vi "Get Curve Limitation.vi"(8 "error in (no error)":errorcluster, 11 "ProductNum":string) -> (0 "error out":errorcluster, 1 "X data Range":dbl[](array[numeric]), 2 "Kb":T1, 3 "Up down Limit XY array":cluster{dbl[], "Xt resampled":dbl[]}[](array[cluster]))   [LabVIEW 2015, in "SQLite.lvclass"]
doc: "写入每一步的测试结果到Results表格。\n写入原理：先检测已经保存了几个结果数据，然后依次附加到结果数据列上。\n# 2020-6-8 14:05:45"
uses:
  SQLite.lvclass
  TwoPoint Curve Limitation Kb.ctl
  SQLiteFileName.ctl
  TabelFullName.ctl
  <vilib>/Utility/error.llb/Trim Whitespace.vi
  <vilib>/addons/Time Series Analysis/Series Preprocess.llb/TSA Resampling (Equal).vi
  <userlib>/sushu/sushu.lvlib
  <vilib>/addons/_Advanced Signal Processing/NI_AdvSigProcTSA.lvlib
panel:
  out "XY Graph":cluster{dbl[], dbl[]}[](graph)
  out "appended array 2":dbl[](array[numeric])
  out "appended array":dbl[](array[numeric])
  in  "Results List":string
  out "CMD":string
  in  "StationName":string
  out "number (0 to 1)":dbl
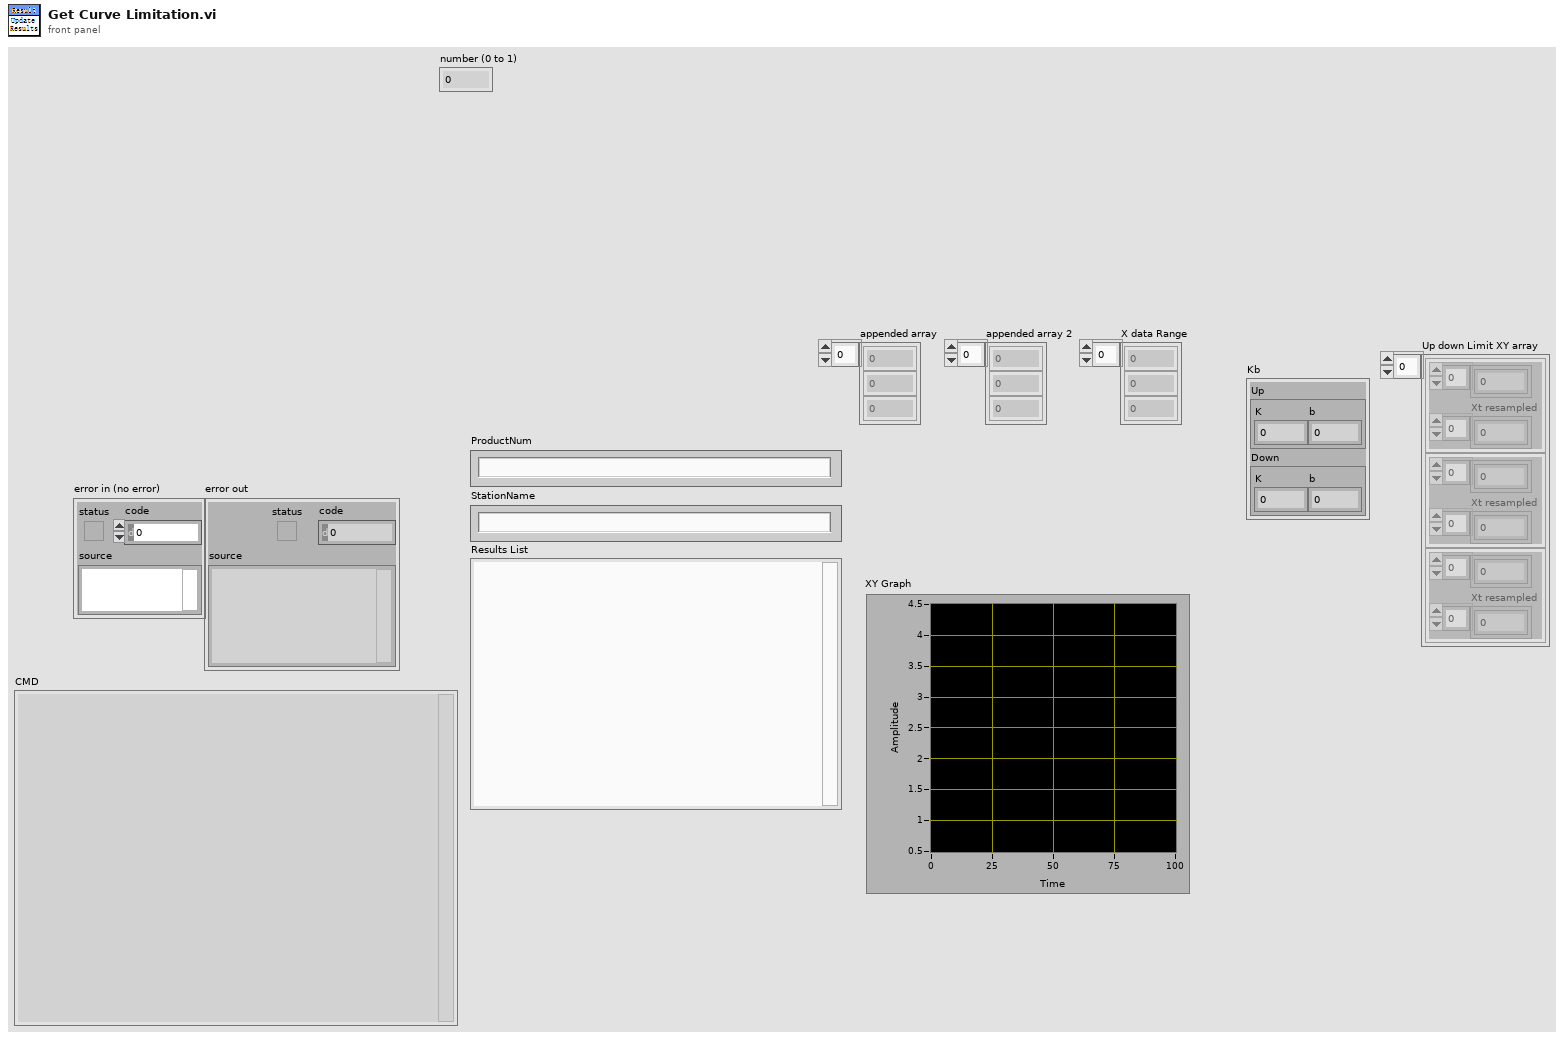
[diagram p1: front panel]
types:
  T1 = typedef "SQLite.lvclass/TwoPoint Curve Limitation Kb.ctl" = cluster{"Up":cluster{"K":dbl, "b":dbl}, "Down":cluster{"K":dbl, "b":dbl}}
  T2 = typedef "SQLite.lvclass/TabelFullName.ctl" = string
  T3 = typedef "SQLite.lvclass/SQLiteFileName.ctl" = string
  T4 = cluster{"Core":cluster{"Current VI Reference":refnum<vi>, "Close Panel on Exit?":bool}, "VI Name":string, "Row Numbers":string, "Update?":bool, "CMD":string, "ResultStartindex":i32, "EmptyResultColumnIndex":i32, "Kb":T1}
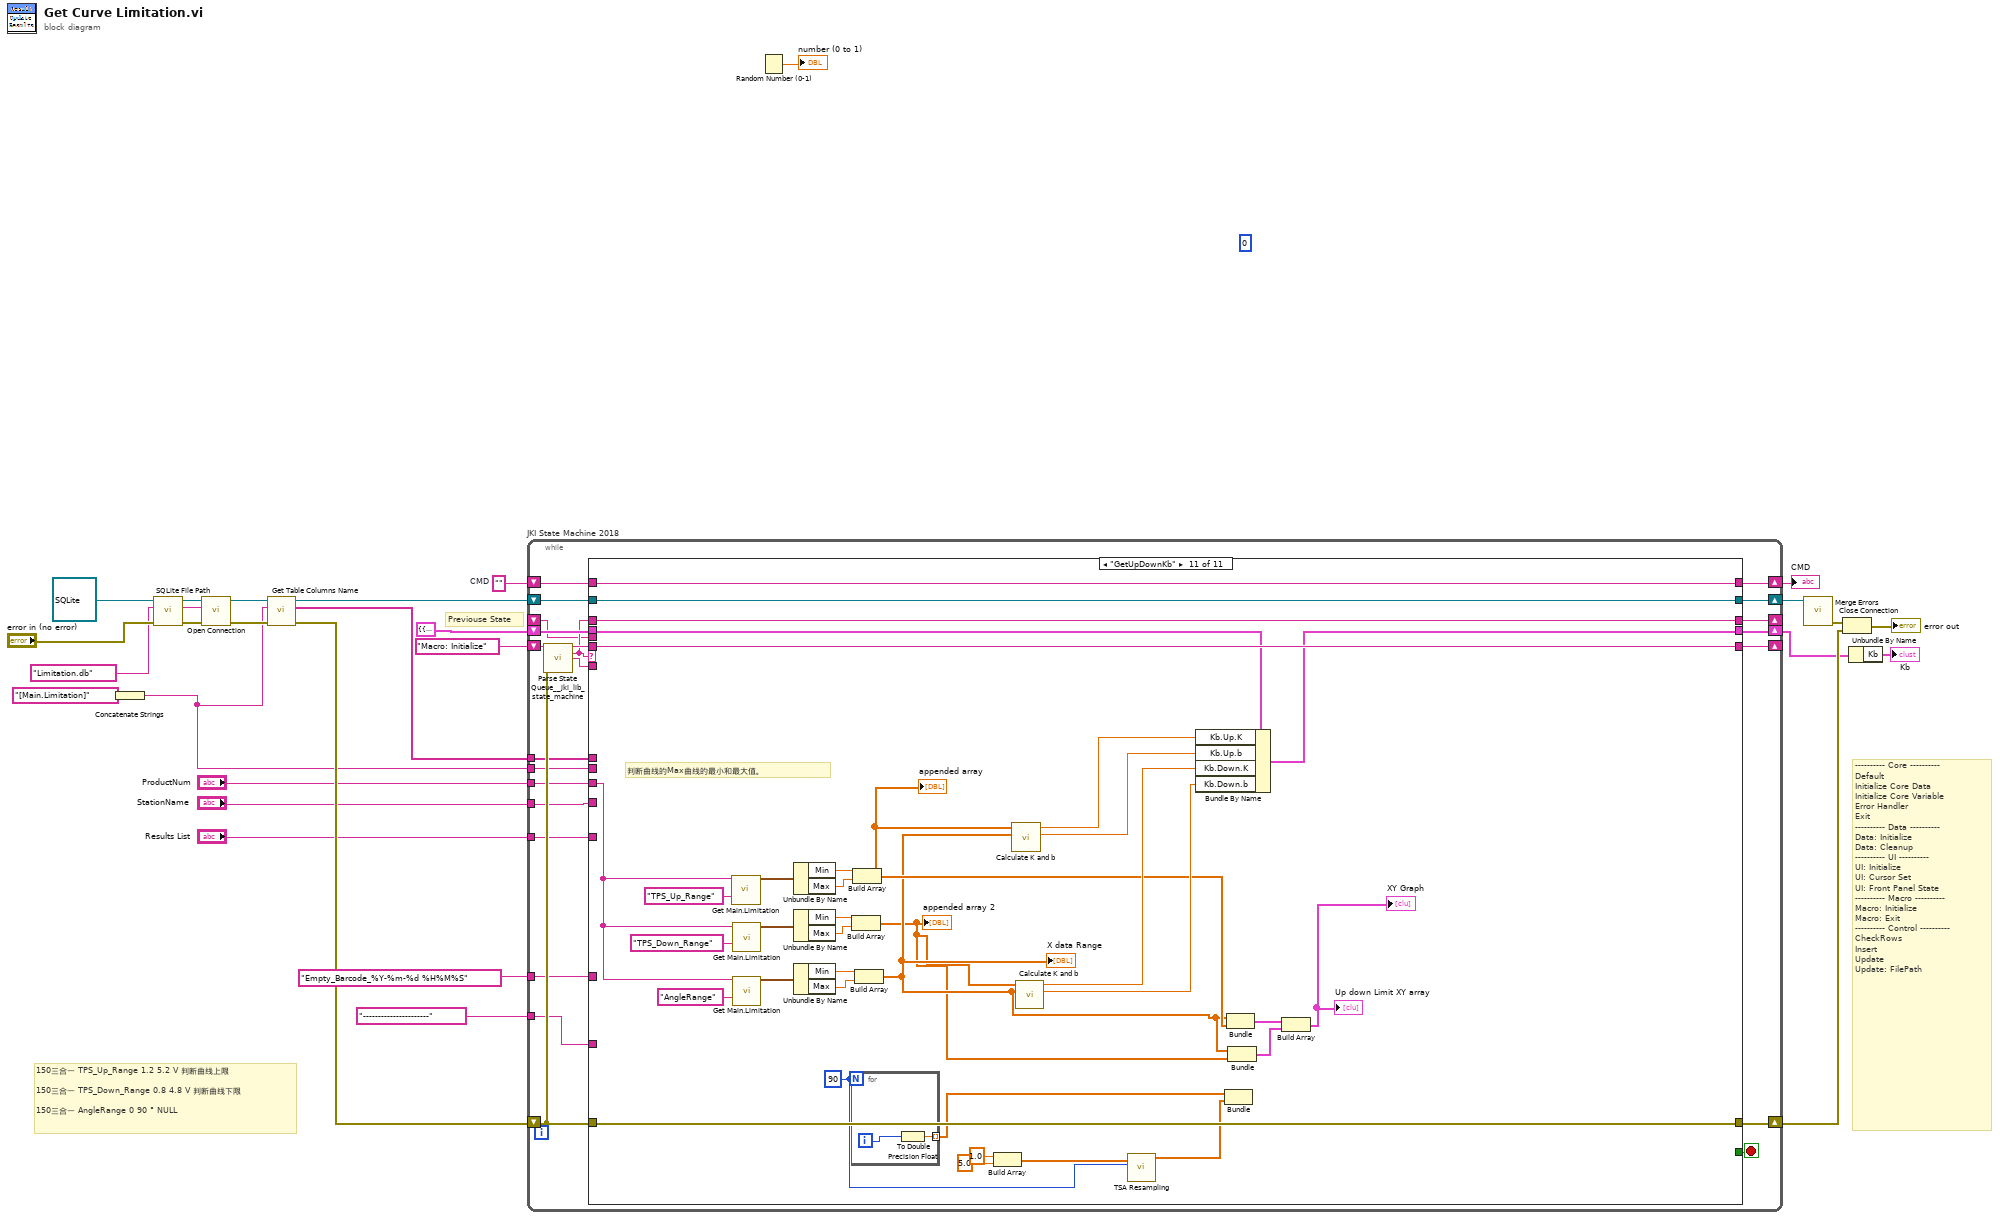
[diagram p0: block diagram]
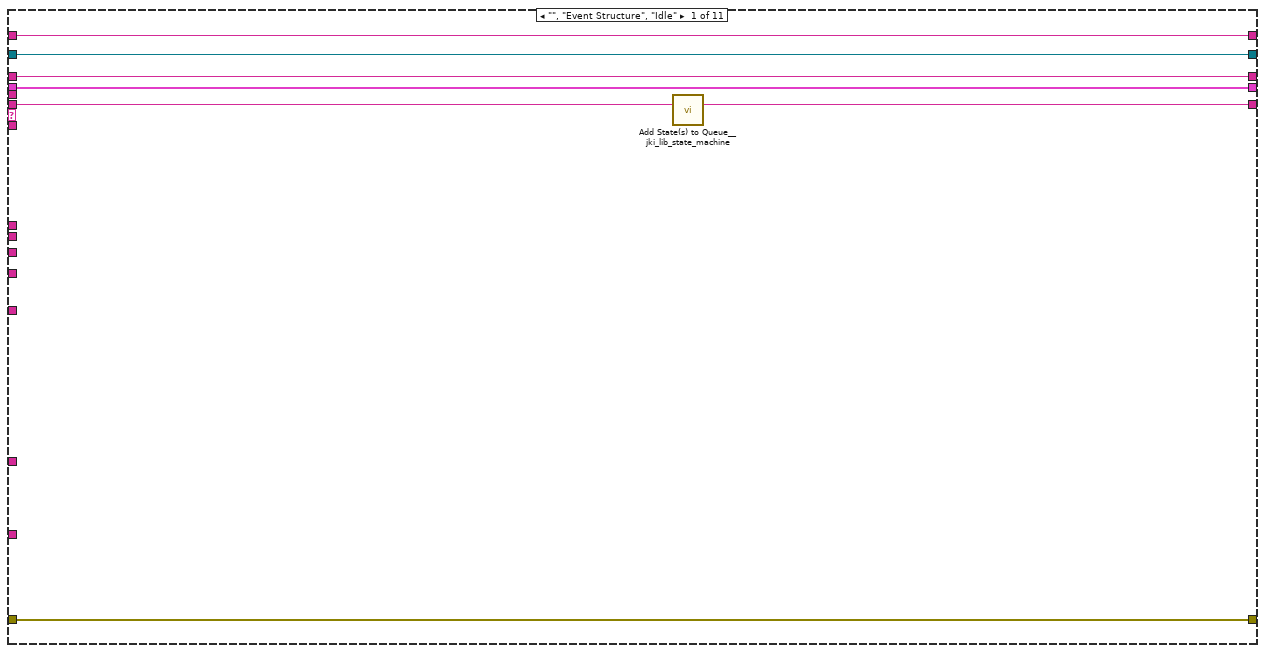
[diagram p2: hidden frame]
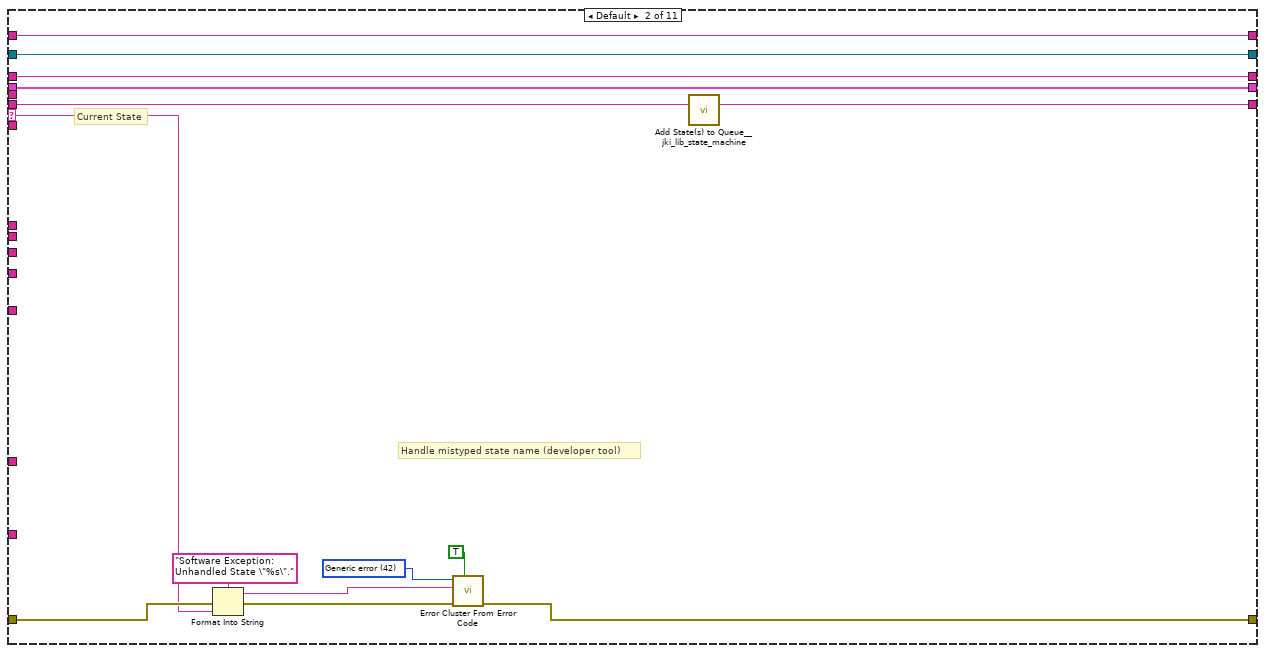
[diagram p3: hidden frame]
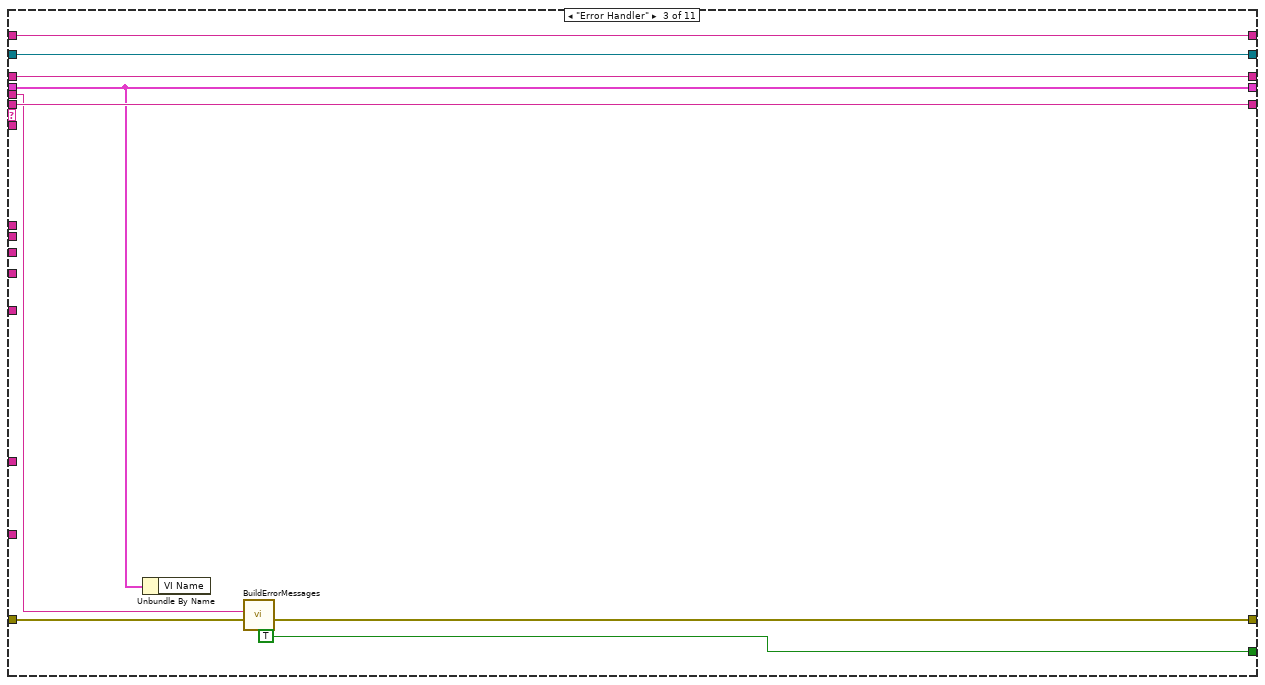
[diagram p4: hidden frame]
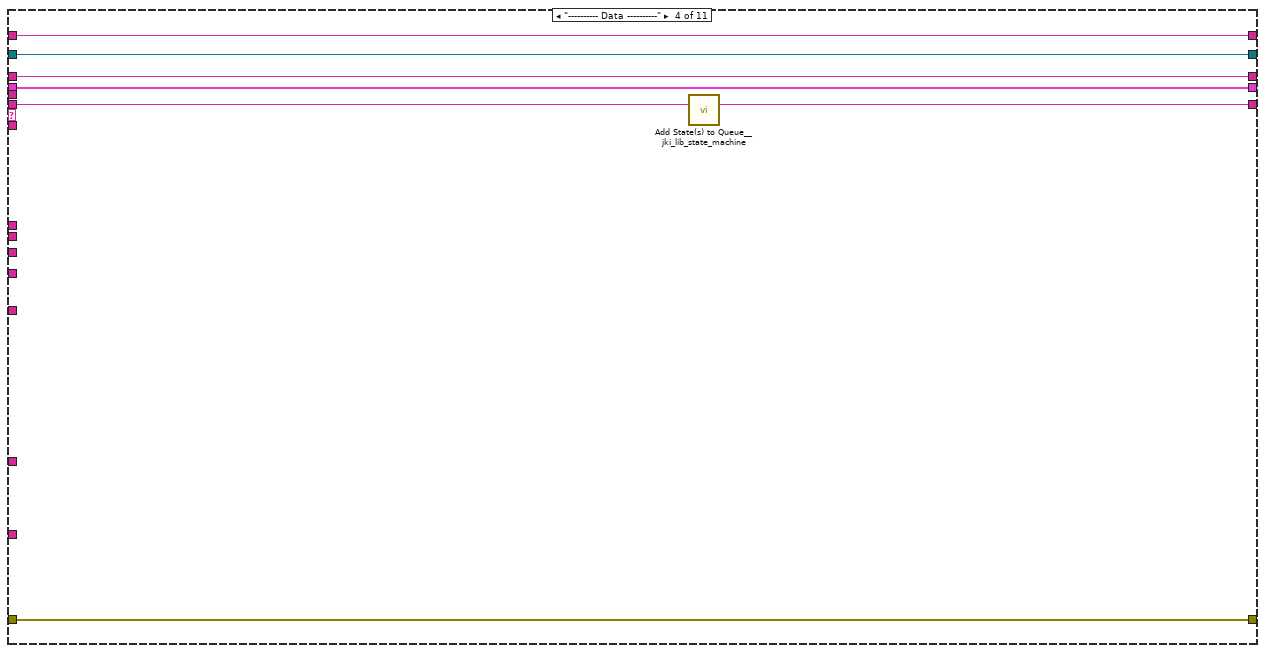
[diagram p5: hidden frame]
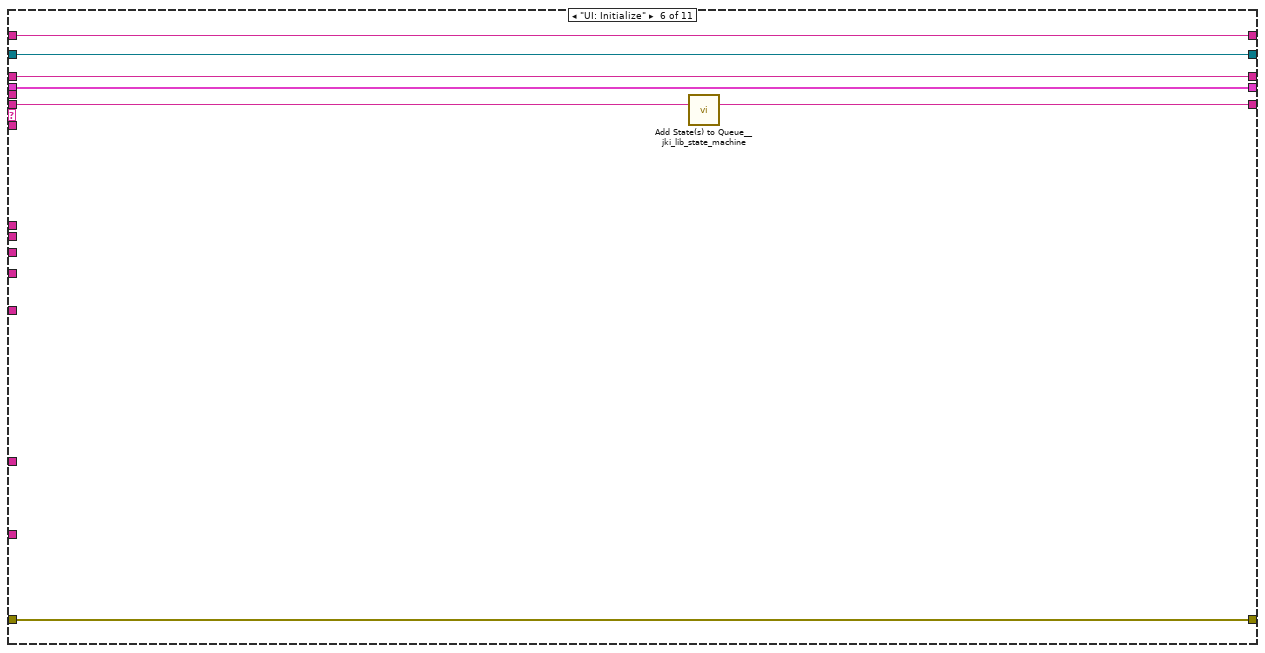
[diagram p7: hidden frame]
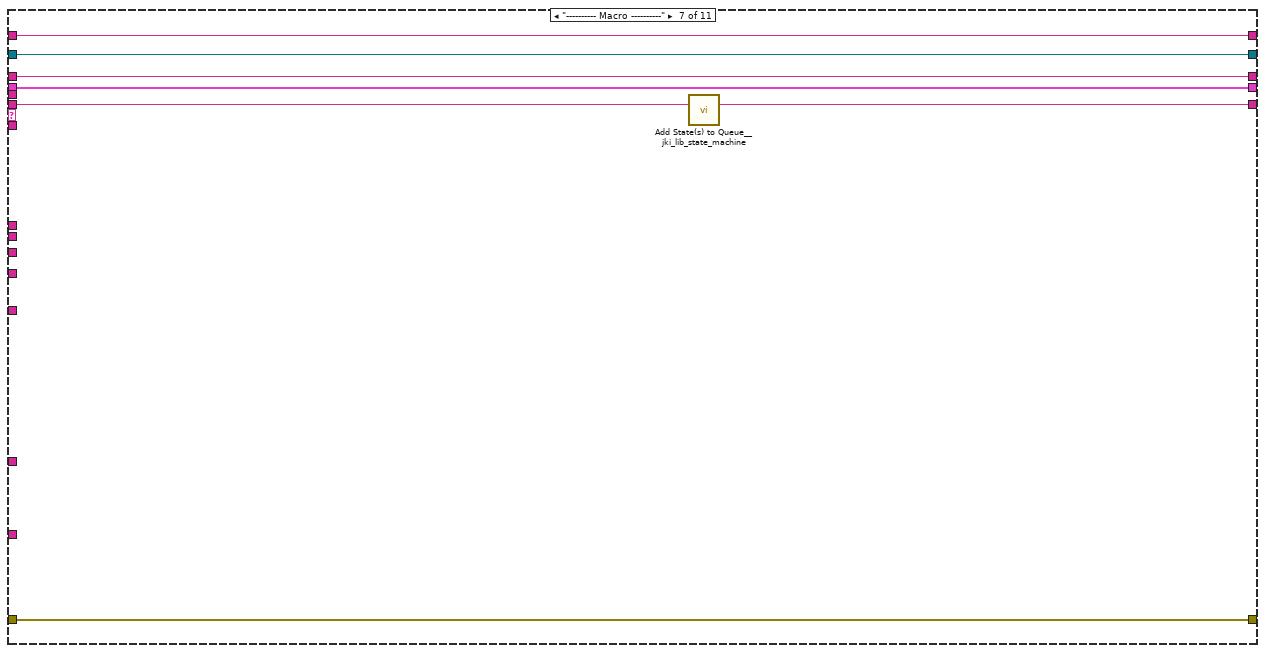
[diagram p8: hidden frame]
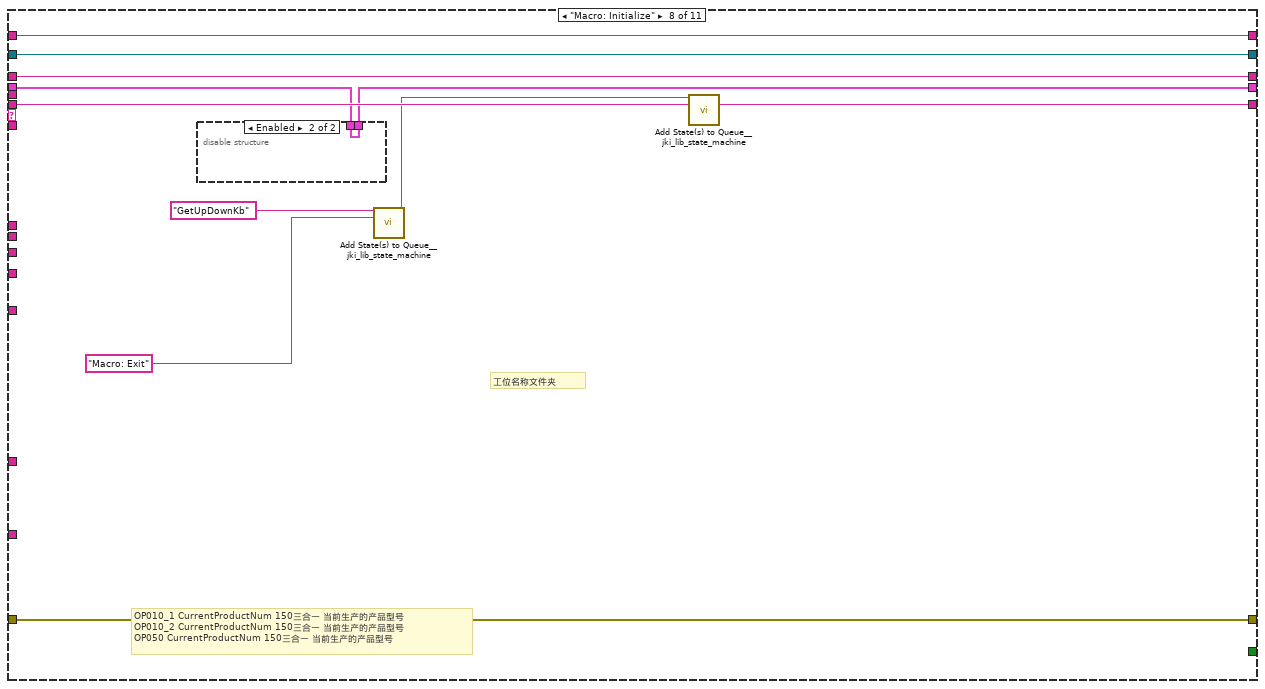
[diagram p9: hidden frame]
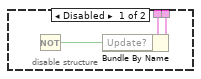
[diagram p10: hidden frame]
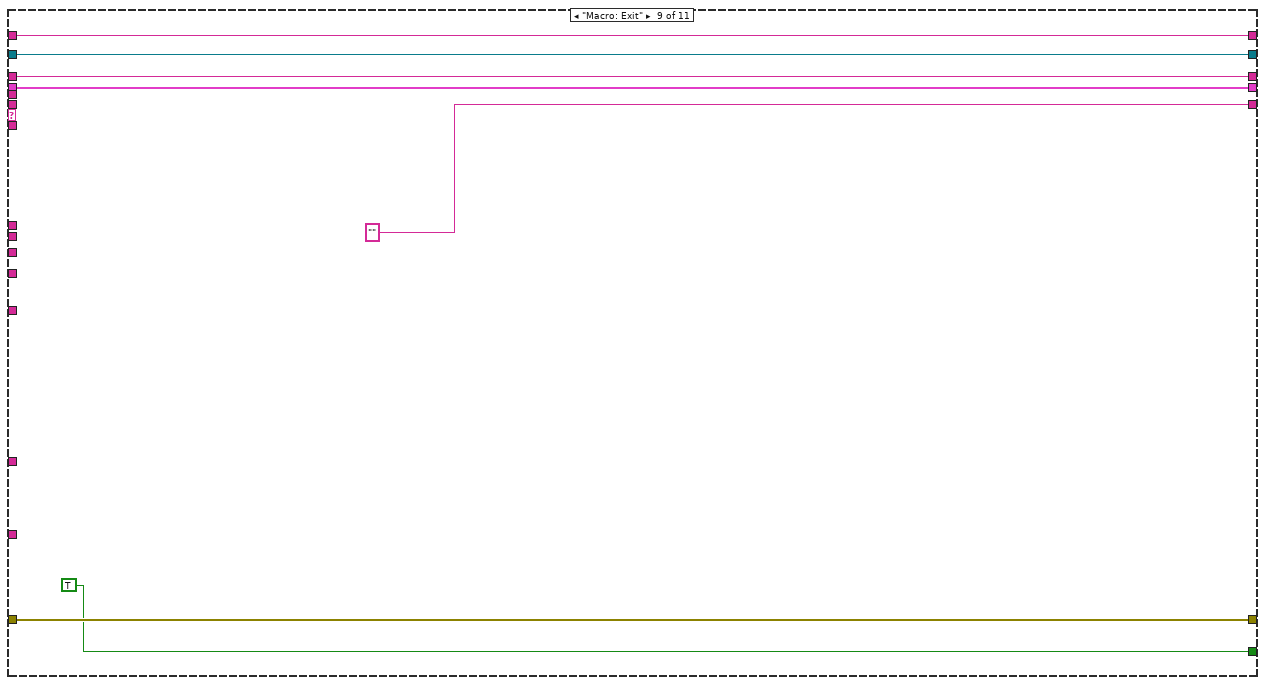
[diagram p11: hidden frame]
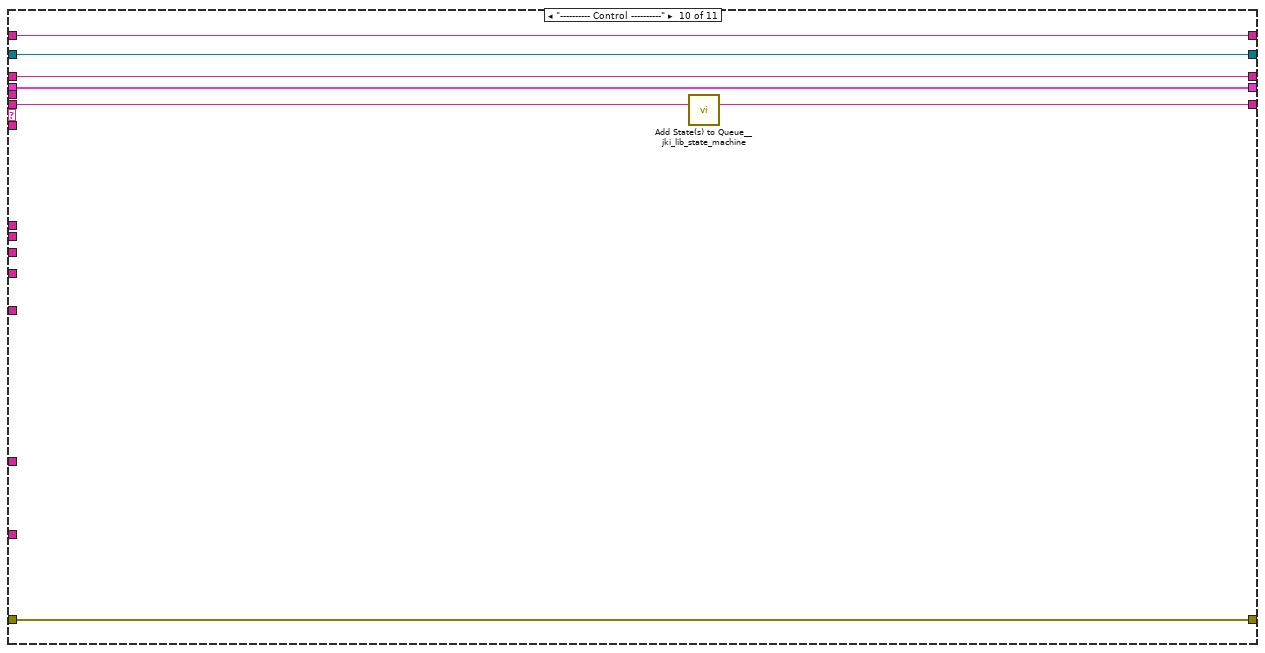
[diagram p12: hidden frame]
diagram:
  w14 = ""  # CMD
  (unwired) 0 ("index (row)")
  # "150三合一\tTPS_Up_Range\t1.2\t5.2\tV\t判断曲线上限\n\n150三合一\tTPS_Down_Range\t0.8\t4.8\tV\t判断曲线下限\n\n150三合一\tAngleRange\t0\t90\t°\tNULL"
  # "Previouse State"
  # "---------- Core ----------\nDefault\nInitialize Core Data\nInitialize Core Variable\nError Handler\nExit\n---------- Data ----------\nData: Initialize\nData: Cleanup\n---------- UI ----------\nUI: Initialize\nUI: Cursor Set\nUI: Front Panel State\n---------- Macro ----------\nMacro: Initialize\nMacro: Exit\n---------- Control ----------\nCheckRows\nInsert\nUpdate\nUpdate: FilePath"
  n1 = Concatenate Strings(T2 "[Main.Limitation]" ("TabelFullName")) -> (w3:string)
  n2 = call "SQLite File Path.vi"("error in (no error)"="error in (no error)", "SQLiteFileName"=T3 "Limitation.db", "SQLite in"=refnum<class "SQLite.lvclass"> refnum ("SQLite.lvclass")) -> ("error out"=w6:errorcluster, "string"=w10:string, "SQLite out"=w8:refnum<class "SQLite.lvclass">)  [unwired: 6 in]
  n3 = call-dynamic "Open Connection.vi"("error in (no error)"=w6, "ConnectionString"=w10, "HostDB in"=w8) -> ("error out"=w27:errorcluster, "HostDB out"=w28:refnum<class "SQLite.lvclass">)  [unwired: 7 in]
  n4 = call-dynamic "Get Table Columns Name.vi"("error in (no error)"=w27, "TableName"=w3, "HostDB in"=w28) -> ("error out"=w19:errorcluster, "ColunmsList"=w18:string[], "HostDB out"=w23:refnum<class "SQLite.lvclass">)  [unwired: 4 in, 2 out]
  n5 = while "JKI State Machine 2018" {
    shift-right: [w46] -> w2
    shift-left: T4 {"Core"={"Current VI Reference"=refnum, "Close Panel on Exit?"=FALSE}, "VI Name"="", "Row Numbers"="", "Update?"=FALSE, "CMD"="", "ResultStartindex"=0, "EmptyResultColumnIndex"=0, "Kb"={"Up"={"K"=0.0, "b"=0.0}, "Down"={"K"=0.0, "b"=0.0}}} ("Data") -> [w45]
    shift-right: [w49] -> w20
    shift-left: w19 -> [w44]
    shift-right: [w48] -> _
    shift-left: "Macro: Initialize" -> [w50]
    shift-right: [w42] -> w22
    shift-left: w23 -> [w43]
    shift-right: [w40] -> _
    shift-left: _ -> [w39]
    tunnel: "StationName" -> [w38]
    tunnel: "ProductNum" -> [w37]
    tunnel: w18 -> [w36]
    tunnel: w3 -> [w35]
    tunnel: "Empty_Barcode_%Y-%m-%d %H%M%S" ("time format string (%c)") -> [w34]
    shift-right: [w33] -> w12
    shift-left: w14 -> [w32]
    tunnel: "----------------------" ("State(s) in (\"\")") -> [w31]
    tunnel: "Results List" -> [w30]
    stop <- w47 stop-if-true
    n6 = call <vilib>:"Parse State Queue__jki_lib_state_machine.vi"("State Queue"=w50, "Error In (no error)"=w44) -> ("Remaining States"=w52:string, "Current State"=w41:string, "Arguments"=w51:string)  [unwired: 11 in]
    n7 = case shown="\"GetUpDownKb\"" w41 {
      selector: w41 -> [_ w63 _ _ _ _ _ _ _ _ _]
      tunnel: w52 -> [w59 w67 w81 w89 w92 w102 w109 w120 _ w138 w173]
      tunnel: w51 -> [_ _ _ _ _ _ _ _ _ _ _]
      tunnel: w45 -> [w56 w65 w78 w86 w93 w100 w106 w115 w130 w135 w152]
      tunnel: [w57 w69 w75 w87 w95 w99 w107 w116 w131 w136 w174] -> w49
      tunnel: w44 -> [w57 w68 w76 w87 w95 w99 w107 w116 w131 w136 w174]
      tunnel: [w58 w66 w81 w88 w92 w101 w108 w119 "" w137 w173] -> w48
      tunnel: [_ _ TRUE _ _ _ _ _ TRUE _ _] -> w47
      tunnel: [w56 w65 w78 w86 w93 w100 w106 w111 w130 w135 w151] -> w46
      tunnel: w43 -> [w55 w62 w80 w85 w94 w98 w105 w118 w129 w134 w172]
      tunnel: [w55 w62 w80 w85 w94 w98 w105 w118 w129 w134 w172] -> w42
      tunnel: w41 -> [w54 w61 w79 w84 w91 w97 w104 w117 w127 w133 w171]
      tunnel: [w54 w61 w79 w84 w91 w97 w104 w117 w127 w133 w171] -> w40
      tunnel: w39 -> [_ _ w77 _ _ _ _ _ _ _ _]
      tunnel: w38 -> [_ _ _ _ _ _ _ _ _ _ _]
      tunnel: w37 -> [_ _ _ _ _ _ _ _ _ _ w166]
      tunnel: w36 -> [_ _ _ _ _ _ _ _ _ _ _]
      tunnel: w35 -> [_ _ _ _ _ _ _ _ _ _ _]
      tunnel: w34 -> [_ _ _ _ _ _ _ _ _ _ _]
      tunnel: w32 -> [w53 w60 w74 w83 w90 w96 w103 w112 w125 w132 w170]
      tunnel: [w53 w60 w74 w83 w90 w96 w103 w112 w125 w132 w170] -> w33
      tunnel: w31 -> [_ _ _ _ _ _ _ _ _ _ _]
      tunnel: w30 -> [_ _ _ _ _ _ _ _ _ _ _]
      frame "", "Event Structure", "Idle" {
        n8 = call <vilib>:"Add State(s) to Queue__jki_lib_state_machine.vi"("State(s) in (\"\")"=w59) -> ("States Out"=w58:string)  [unwired: 14 in]
      }
      frame Default {
        w72 = 42 items=["No error", "Argument error", "Memory is full", "Out of zone", "End of file", "File already open", "Generic file I/O error", "File not found", "File permission error", "Disk is full", "Duplicate path", "Too many files open", "System feature not enabled", "Resource file not found", "Cannot add resource", "Resource not found", "Image not found", "Image memory error", "Pen does not exist", "Config type invalid", "Config token not found", "Config parse error", "Config memory error", "Bad external code format", "Bad external code offset", "External code not present", "Null window", "Destroy window error", "Null menu", "Print aborted", "Bad print record", "Print driver error", "Windows error during printing", "Memory error during printing", "Print dialog error", "Generic print error", "Invalid device refnum", "Device not found", "Device parameter error", "Device unit error", "Cannot open device", "Device call aborted", "Generic error", "Cancelled by user", "Object ID too low", "Object ID too high", "Object not in heap", "Unknown heap", "Unknown object (invalid DefProc)", "Unknown object (DefProc not in table)", "Message out of range", "Invalid (null) method", "Unknown message", "Manager call not supported", "Bad address", "Network operation in progress", "Network operation timed out", "Connection is busy", "Network attribute not supported", "Network error", "Address in use", "System out of memory", "Connection aborted", "Connection refused", "Not connected", "Already connected", "Connection closed", "Initialization error (interapplication manager)", "Bad occurrence", "Wait on unbound occurrence handler", "Occurrence queue overflow", "Datalog type conflict", "Unused", "Unrecognized type (interapplication manager)", "Memory corrupt", "Failed to make temporary DLL", "Old CIN version", "Drag socket not found", "Failed to load drop-object", "Failed to register OLE object", "Failed to release OLE object", "Format specifier type mismatch", "Unknown format specifier", "Too few format specifiers", "Too many format specifiers", "Scan failed", "Newer CIN version", "Error converting to variant", "Runtime menu error", "Password tampered", "Variant attribute not found", "Incompatible variant data type", "Event data is not available", "Event Store is not present", "Occurrence is not found", "Event Queue is not created", "Event info is not available", "Refnum passed is NULL", "Error retrieving Class GUID", "Error retrieving CoClass GUID", "Error retrieving TypeLib GUID.", "Bad built application magic bytes.", "Specific driver is different from the specific driver associated with the Logical Name.", "There is no session opened to the class driver.", "Max Error", "MAX - Error with config objects", "MAX - Error loading configuration", "MAX - Group not supported"]
        # "Current State"
        # "Handle mistyped state name (developer tool)"
        n9 = Format Into String(format string="Software Exception: Unhandled State \"%s\"." ("message"), error in=w68, w63) -> (resulting string=w71:string, error out=w70:errorcluster)  [unwired: 1 in]
        n10 = call <vilib>:"Error Cluster From Error Code.vi"("show call chain? (False)"=TRUE, "error in (no error)"=w70, "error message (\"\")"=w71, "error code (0)"=w72) -> ("error out"=w69:errorcluster)  [unwired: 5 in]
        n11 = call <vilib>:"Add State(s) to Queue__jki_lib_state_machine.vi"("State(s) in (\"\")"=w67) -> ("States Out"=w66:string)  [unwired: 14 in]
      }
      frame "Error Handler" {
        n12 = Unbundle By Name(w78) -> ()  [unwired: 1 out]
        n13 = call <userlib>:"BuildErrorMessages.vi"("error in"=w76, "ErrorCase"=w77) -> ("error out (no error)"=w75:errorcluster)  [unwired: 7 in, 2 out]
      }
      frame "---------- Data ----------" {
        n14 = call <vilib>:"Add State(s) to Queue__jki_lib_state_machine.vi"("State(s) in (\"\")"=w89) -> ("States Out"=w88:string)  [unwired: 14 in]
      }
      frame "Data: Initialize" {
      }
      frame "UI: Initialize" {
        n15 = call <vilib>:"Add State(s) to Queue__jki_lib_state_machine.vi"("State(s) in (\"\")"=w102) -> ("States Out"=w101:string)  [unwired: 14 in]
      }
      frame "---------- Macro ----------" {
        n16 = call <vilib>:"Add State(s) to Queue__jki_lib_state_machine.vi"("State(s) in (\"\")"=w109) -> ("States Out"=w108:string)  [unwired: 14 in]
      }
      frame "Macro: Initialize" {
        # "OP010_1\tCurrentProductNum\t150三合一\t当前生产的产品型号\nOP010_2\tCurrentProductNum\t150三合一\t当前生产的产品型号\nOP050\tCurrentProductNum\t150三合一\t当前生产的产品型号"
        # "工位名称文件夹"
        n17 = disable-structure shown="Enabled" {
          disable-tunnel: w115 -> [w123 w124]
          disable-tunnel: [w122 w124] -> w111
          frame Disabled {
            n18 = Not() -> (.not. x?=w121:bool)  [unwired: 1 in]
            n19 = Bundle By Name(cluster=w123, "Update?"=w121) -> (w122:T4)
          }
          frame Enabled {
          }
        }
        n20 = call <vilib>:"Add State(s) to Queue__jki_lib_state_machine.vi"("State(s) in Front (\"\")"="GetUpDownKb" ("State(s) in Front (\"\")"), "State(s) in (\"\")"="Macro: Exit") -> ("States Out"=w114:string)  [unwired: 13 in]
        n21 = call <vilib>:"Add State(s) to Queue__jki_lib_state_machine.vi"("State(s) in Front (\"\")"=w114, "State(s) in (\"\")"=w120) -> ("States Out"=w119:string)  [unwired: 13 in]
      }
      frame "Macro: Exit" {
      }
      frame "---------- Control ----------" {
        n22 = call <vilib>:"Add State(s) to Queue__jki_lib_state_machine.vi"("State(s) in (\"\")"=w138) -> ("States Out"=w137:string)  [unwired: 14 in]
      }
      frame "GetUpDownKb" {
        w141 = 90
        # "判断曲线的Max曲线的最小和最大值。"
        n23 = call "Get Main.Limitation.vi"("Main"=w166, "VariableName"="TPS_Up_Range") -> ("Data-DBL"=w165:cluster{"Max":dbl, "Min":dbl})  [unwired: 8 in, 5 out]
        n24 = call "Get Main.Limitation.vi"("Main"=w166, "VariableName"="TPS_Down_Range") -> ("Data-DBL"=w157:cluster{"Max":dbl, "Min":dbl})  [unwired: 8 in, 5 out]
        n25 = call "Get Main.Limitation.vi"("Main"=w166, "VariableName"="AngleRange") -> ("Data-DBL"=w160:cluster{"Max":dbl, "Min":dbl})  [unwired: 8 in, 5 out]
        n26 = Unbundle By Name(w165) -> ("Min"=w164:dbl, "Max"=w163:dbl)
        n27 = Unbundle By Name(w157) -> ("Min"=w159:dbl, "Max"=w158:dbl)
        n28 = Unbundle By Name(w160) -> ("Min"=w161:dbl, "Max"=w162:dbl)
        n29 = for {
          N: w141 -> [_]
          tunnel: [w175] -> w140 mode=indexing
          i -> [w176]
          n30 = To Double Precision Float(number=w176) -> (double precision float=w175:dbl)
        }
        n31 = Build Array(w159, w158) -> (w148:dbl[])
        "appended array 2" <- w148
        n32 = Build Array(w164, w163) -> (w150:dbl[])
        "appended array" <- w150
        n33 = Build Array(w161, w162) -> (w149:dbl[])
        "X data Range" <- w149
        n34 = Build Array(1.0 ("element"), 5.0 ("element")) -> (w142:dbl[])
        n35 = call "Calculate K and b.vi"("X"=w149, "Y"=w150) -> ("b"=w155:dbl, "K"=w156:dbl)  [unwired: 8 in]
        n36 = call "Calculate K and b.vi"("X"=w149, "Y"=w148) -> ("b"=w153:dbl, "K"=w154:dbl)  [unwired: 8 in]
        n37 = call-poly <vilib>:"TSA Resampling.vi"("new sampling rate"=w141, "Xt"=w142) -> ("Xt resampled"=w139:dbl[])  [unwired: 8 in, 1 out]
        n38 = Bundle By Name(cluster=w152, "Kb.Up.K"=w156, "Kb.Up.b"=w155, "Kb.Down.K"=w154, "Kb.Down.b"=w153) -> (w151:T4)
        n39 = Bundle(w140, "Xt resampled"=w139) -> ()  [unwired: 1 in, 1 out]
        n40 = Bundle(w149, w150) -> (w147:cluster{dbl[], dbl[]})  [unwired: 1 in]
        n41 = Bundle(w149, w148) -> (w146:cluster{dbl[], dbl[]})  [unwired: 1 in]
        n42 = Build Array(w147, w146) -> (→"XY Graph" →"Up down Limit XY array":cluster{dbl[], dbl[]}[])
      }
    }
  }
  "CMD" <- w12
  n43 = Random Number (0-1)() -> (number: 0 to 1=→"number (0 to 1)":dbl)
  n44 = call-dynamic "Close Connection.vi"("HostDB in"=w22) -> ("error out"=w26:errorcluster)  [unwired: 9 in, 1 out]
  n45 = Merge Errors(w26, w20) -> (→"error out":errorcluster)
  n46 = Unbundle By Name(w2) -> ("Kb"=→"Kb":T1)
